vi "test Copy To Larger Destinationvi.vi"(8 "error in (no error)":errorcluster, 11 "TestCase in":refnum<class "Data Manipulation Tests.lvclass">) -> (0 "error out":errorcluster, 3 "TestCase out":refnum<class "Data Manipulation Tests.lvclass">)   [LabVIEW 2020, in "Memory Manager Tests.lvlib" / "Data Manipulation Tests.lvclass"]
uses:
  Data Manipulation Tests.lvclass
  Source/Classes/Pointer/Write 1D I32.vi
  Source/Classes/Pointer/Read 1D I32.vi
  <vilib>/addons/_JKI Toolkits/VI Tester/TestCase.llb/TestCase.lvclass
  Source/Classes/Pointer/Pointer.lvclass
  C:/Program Files (x86)/National Instruments/LabVIEW 2020/vi.lib/addons/_JKI Toolkits/VI Tester/TestCase.llb/TestCase.lvclass
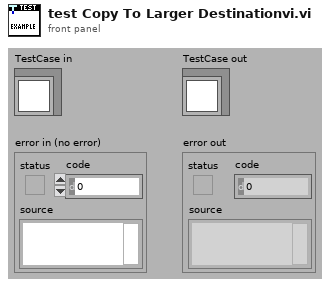
[diagram p1: front panel]
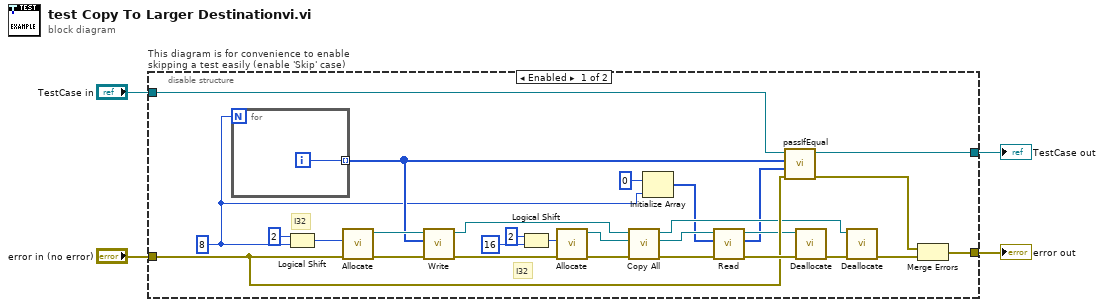
[diagram p0: block diagram]
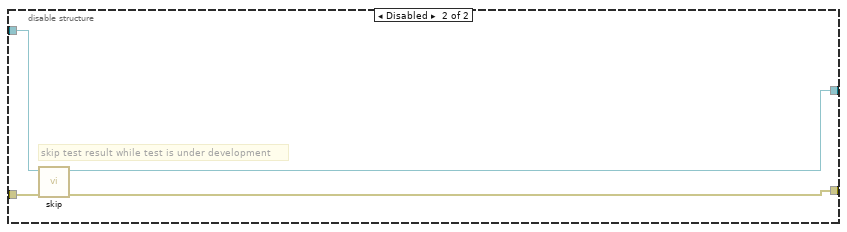
[diagram p2: hidden frame]
diagram:
  n1 = disable-structure "This diagram is for convenience to enable skipping a test easily (enable 'Skip' case)" shown="Enabled" {
    disable-tunnel: "TestCase in" -> [w24 w37]
    disable-tunnel: [w23 w35] -> w1
    disable-tunnel: [w27 w36] -> w3
    disable-tunnel: "error in (no error)" -> [w18 w34]
    frame Enabled {
      w10 = u64 8 ("count (1)")
      # "I32"
      # "I32"
      n2 = for {
        N: w10 -> [_]
        tunnel: [w33] -> w16 mode=indexing
        i -> [w33]
      }
      n3 = Logical Shift(y=i16 2, x=w10) -> (x << y=w9:u64)
      n4 = call "Allocate.vi"("error in (no error)"=w18, "size"=w9) -> ("error out"=w30:errorcluster, "Pointer out"=w32:refnum<class "Pointer.lvclass">)  [unwired: 8 in]
      n5 = call-poly "Write.vi"("error in (no error)"=w30, "buffer in"=w16, "Pointer in"=w32) -> ("error out"=w29:errorcluster, "Pointer out"=w6:refnum<class "Pointer.lvclass">)  [unwired: 5 in, 2 out]
      n6 = Logical Shift(y=i16 2, x=u64 16 ("count (1)")) -> (x << y=w7:u64)
      n7 = call "Allocate.vi"("error in (no error)"=w29, "size"=w7) -> ("error out"=w28:errorcluster, "Pointer out"=w31:refnum<class "Pointer.lvclass">)  [unwired: 8 in]
      n8 = call "Copy All.vi"("error in (no error)"=w28, "dst Pointer in"=w31, "src Pointer in"=w6) -> ("error out"=w21:errorcluster, "dst Pointer out"=w25:refnum<class "Pointer.lvclass">, "src Pointer out"=w13:refnum<class "Pointer.lvclass">)  [unwired: 6 in]
      n9 = Initialize Array(0 ("element"), w10) -> (w12:i32[])
      n10 = call-poly "Read.vi"("error in (no error)"=w21, "buffer in"=w12, "Pointer in"=w25) -> ("error out"=w20:errorcluster, "buffer out"=w11:i32[], "Pointer out"=w17:refnum<class "Pointer.lvclass">)  [unwired: 5 in, 1 out]
      n11 = call-dynamic "passIfEqual.vi"("error in (no error)"=w18, "y"=w11, "x"=w16, "TestCase in"=w24) -> ("error out"=w19:errorcluster, "TestCase out"=w23:refnum<class "Data Manipulation Tests.lvclass">)  [unwired: 6 in]
      n12 = call "Deallocate.vi"("error in (no error)"=w20, "Pointer"=w17) -> ("error out"=w15:errorcluster)  [unwired: 8 in, 1 out]
      n13 = call "Deallocate.vi"("error in (no error)"=w15, "Pointer"=w13) -> ("error out"=w14:errorcluster)  [unwired: 8 in, 1 out]
      n14 = Merge Errors(w19, w14) -> (w27:errorcluster)
    }
    frame Disabled {
      # "skip test result while test is under development"
      n15 = call <vilib>:"skip.vi"("error in (no error)"=w34, "TestCase in"=w37) -> ("error out"=w36:errorcluster, "TestCase out"=w35:refnum<class "Data Manipulation Tests.lvclass">)  [unwired: 8 in]
    }
  }
  "error out" <- w3
  "TestCase out" <- w1
